vi "Periodic Tasks.vi"(8 "error constant":errorcluster) -> ()   [LabVIEW 2014]
doc: "This VI runs in parallel to other tasks. It can contain as many user-defined periodic loops as you need. These can carry out PID or other sorts of timed response."
uses:
  <vilib>/Rock Robotics/WPI/Relay/WPI_RelayValue.ctl
  <vilib>/Rock Robotics/WPI/Solenoid/WPI_SolenoidValue.ctl
  <vilib>/Rock Robotics/WPI/Compressor/WPI_CompressorGetSetRefNum.vi
  <vilib>/Rock Robotics/WPI/RobotDrive/WPI_RobotDriveGetSetRefNum.vi
  Robot Global Data.vi
  <vilib>/Rock Robotics/WPI/RobotDrive/WPI_RobotDriveMecanumDrive_Cartesian.vi
  <vilib>/addons/control/pid/pid.llb/PID (DBL).vi
  navX-MXP Library/navX-MXP IMU.lvlib
  <vilib>/addons/control/pid/NI_PID_pid.lvlib
panel:
  out "Voltage 2":dbl
  out "Level Pre Coerce":sgl
  out "String Potentiometer":dbl
  out "Setpoint from Teleop":dbl(slide) scale=3.7..4.5
  in  "SetPoint":dbl(slide) step=0.01 scale=3.7..4.5
  out "Brake":bool
  out "Doors Oper":bool
  out "Grabber":bool
  out "output":dbl format="%.2f"
  out "Voltage":dbl(slide) scale=0.0..5.0
  in  "proportional gain (Kc)":dbl=10.0 step=0.01
  in  "integral time (Ti, min)":dbl=0.001 step=0.01
  in  "derivative time (Td, min)":dbl=0.001 step=0.01
  in  "dt (s)":dbl=-1.0 format="%.3f"
  out "Lifter":bool
  out "Rotation":dbl
  out "Y":dbl
  out "X":dbl
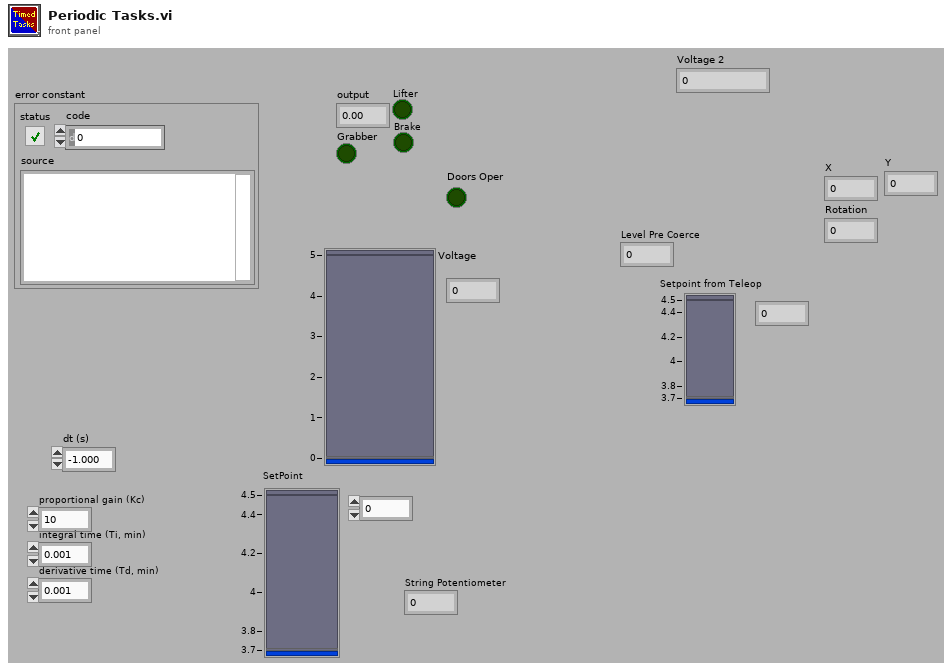
[diagram p1: front panel]
types:
  T1 = typedef "navX-MXP IMU.lvlib/navX SPI DevRef.ctl" = cluster{"SPIDevRef":T2, "Board Information":T5, "Status":T6, "Offsets":cluster{"Yaw":dbl, "Quat W":dbl, "Quat X":dbl, "Quat Y":dbl, "Quat Z":dbl}, "Update Rate (4Hz-60Hz)":u8, "refnum name":string, "error":errorcluster}
  T2 = typedef "WPI_SPIDevRef.ctl" = cluster{"DevStatus":errorcluster, "Handle":i32, "Controller":T3, "SPI Bus":T4}
  T3 = typedef "FPGA_TypedefDigitalModule.ctl" = enum16{"Controller 1"}
  T4 = typedef "spi_bus.ctl" = enum16{"SPI On-Board, CS0", "SPI On-Board, CS1", "SPI On-Board, CS2", "SPI On-Board, CS3", "SPI MXP", "Invalid"}
  T5 = typedef "navX-MXP IMU.lvlib/navX Board Information.ctl" = cluster{"WhoAmI (50 | 0x32)":u8, "Board Revision":u8, "Firmware Major Version":u8, "Firmware Minor Version":u8}
  T6 = typedef "navX-MXP IMU.lvlib/navX Status Data.ctl" = cluster{"Update Rate Hz":u8, "Accelerometer Full-Scale Range":u8, "Gyro Full-Scale Range":u16, "NAVX_OP_STATUS":T7, "NAVX_CAL_STATUS":T8, "NAVX_SELFTEST_STATUS":u8, "NAVX_SENSOR_STATUS":T9}
  T7 = typedef "navX-MXP IMU.lvlib/navX NAVX_OP_STATUS.ctl" = u8
  T8 = typedef "navX-MXP IMU.lvlib/navX NAVX_CAL_STATUS.ctl" = u8
  T9 = typedef "navX-MXP IMU.lvlib/navX NAVX_SENSOR_STATUS.ctl" = cluster{"MOVING":bool, "YAW_STABLE":bool, "MAG_DISTURBANCE":bool, "ALTITUDE_VALID":bool, "SEALEVEL_PRESS_SET":bool, "FUSED_HEADING_VALID":bool}
  T10 = typedef "navX-MXP IMU.lvlib/navX YPRH Data.ctl" = cluster{"Yaw":dbl, "Pitch":dbl, "Roll":dbl, "Heading":dbl}
  T11 = typedef "WPI_SolenoidValue.ctl" = enum16{"Off", "On", "Forward", "Reverse"}
  T12 = cluster{"proportional gain (Kc)":dbl, "integral time (Ti, min)":dbl, "derivative time (Td, min)":dbl}
  T13 = typedef "WPI_MotorControlDeviceRef.ctl" = cluster{"DeviceStatus":errorcluster, "Type":T14, "PWM":cluster{"Controller":T3, "PWM Channel":T15, "DeadBand":T16}, "CAN":cluster{"Device Number":u8, "Control Mode":T17, "Semaphore":T18, "Max Vout":dbl, "TalonSRX Control Mode":T19}, "Invert":bool, "TransformRef":T20, "InvTransformRef":T20}
  T14 = typedef "WPI_MotorControlType.ctl" = enum16{"PWM", "CAN", "CANTalonSRX"}
  T15 = typedef "FPGA_DIOPWMChannel.ctl" = enum8{"PWM 0", "PWM 1", "PWM 2", "PWM 3", "PWM 4", "PWM 5", "PWM 6", "PWM 7", "PWM 8", "PWM 9", "PWM MXP 0", "PWM MXP 1", "PWM MXP 2", "PWM MXP 3", "PWM MXP 4", "PWM MXP 5", "PWM MXP 6", "PWM MXP 7", "PWM MXP 8", "PWM MXP 9", "Invalid"}
  T16 = typedef "WPI_PWMDeadband.ctl" = cluster{"Name":string, "maxPositivePwm":i32, "minPositivePwm":i32, "centerPwm":i32, "maxNegativePwm":i32, "minNegativePwm":i32, "angularRange":u16}
  T17 = typedef "WPI_CANJaguar_ControlMode.ctl" = enum8{"Percent VBus", "Current", "Speed", "Position", "Voltage"}
  T18 = typedef "Semaphore RefNum" = refnum<k1>
  T19 = typedef "WPI_CANTalonSRX_APIControlMode.ctl" = enum8{"Percent VBus", "Speed", "Position", "Slave", "Unchanged / Invalid"}
  T20 = typedef "WPI_PWMTransform_ConPane.ctl" = refnum<vi>
  T21 = typedef "WPI_SolenoidDevRef.ctl" = cluster{"DevStatus":errorcluster, "Pneumatics Control Module":u8, "Forward Solenoid Channel":T22, "Reverse Solenoid Channel":T22}
  T22 = typedef "WPI_SolenoidChannel.ctl" = enum8{"Solenoid 0", "Solenoid 1", "Solenoid 2", "Solenoid 3", "Solenoid 4", "Solenoid 5", "Solenoid 6", "Solenoid 7", "Invalid"}
  T23 = typedef "WPI_AnalogChannelDevRef.ctl" = cluster{"DevStatus":errorcluster, "Controller":T24, "Analog Channel":T25}
  T24 = typedef "FPGA_TypedefAnalogModule.ctl" = enum16{"Controller 1"}
  T25 = typedef "FPGA_AIChannel.ctl" = enum8{"AI 0", "AI 1", "AI 2", "AI 3", "AI MXP 0", "AI MXP 1", "AI MXP 2", "AI MXP 3", "Invalid"}
  T26 = cluster{"Motor Speed":dbl, "Grabber":bool, "Go Up a Level":bool, "Go Down a Level":bool}
  T27 = cluster{"String Potentiometer":dbl, "Setpoint":dbl, "Level":sgl}
  T28 = typedef "WPI_RobotDriveDevRef.ctl" = cluster{"DevStatus":errorcluster, "Motors[]":T13[], "Square Inputs":bool, "Max Output":dbl}
  T29 = typedef "WPI_CompressorDevRef.ctl" = cluster{"DevStatus":errorcluster, "Pneumatics Control Module":u8}
  T30 = typedef "WPI_RelayDevRef.ctl" = cluster{"DevStatus":errorcluster, "Relay Channel":T31, "Controller":T3, "Relay Direction":T32}
  T31 = typedef "FPGA_DIORelayChannel.ctl" = enum8{"Relay 0", "Relay 1", "Relay 2", "Relay 3", "Invalid"}
  T32 = typedef "WPI_RelayDirection.ctl" = enum16{"Both directions", "Forward only", "Reverse only"}
  T33 = typedef "WPI_DigitalInputDevRef.ctl" = cluster{"DevStatus":errorcluster, "DIO Channel":T34, "Controller":T3}
  T34 = typedef "FPGA_DIOChannel.ctl" = enum8{"DIO 0", "DIO 1", "DIO 2", "DIO 3", "DIO 4", "DIO 5", "DIO 6", "DIO 7", "DIO 8", "DIO 9", "DIO MXP 0", "DIO MXP 1", "DIO MXP 2", "DIO MXP 3", "DIO MXP 4", "DIO MXP 5", "DIO MXP 6", "DIO MXP 7", "DIO MXP 8", "DIO MXP 9", "DIO MXP 10", "DIO MXP 11", "DIO MXP 12", "DIO MXP 13", "DIO MXP 14", "DIO MXP 15", "Invalid"}
  T35 = typedef "WPI_RelayValue.ctl" = enum16{"Off", "On", "Forward", "Reverse"}
  T36 = cluster{"Lifter Down":bool, "Right Infeed":enum16{"Off", "Forward", "Reverse"}, "Left Infeed":enum16{"Off", "Forward", "Reverse"}}
  T37 = cluster{"Front Right Motor":dbl, "Front Left Motor":dbl, "Rear Right Motor":dbl, "Rear Left Motor":dbl, "Current Heading":dbl, "Tote lift Up":bool, "Feeders Running":bool, "Pressure In Tank":dbl, "Image Data":string}
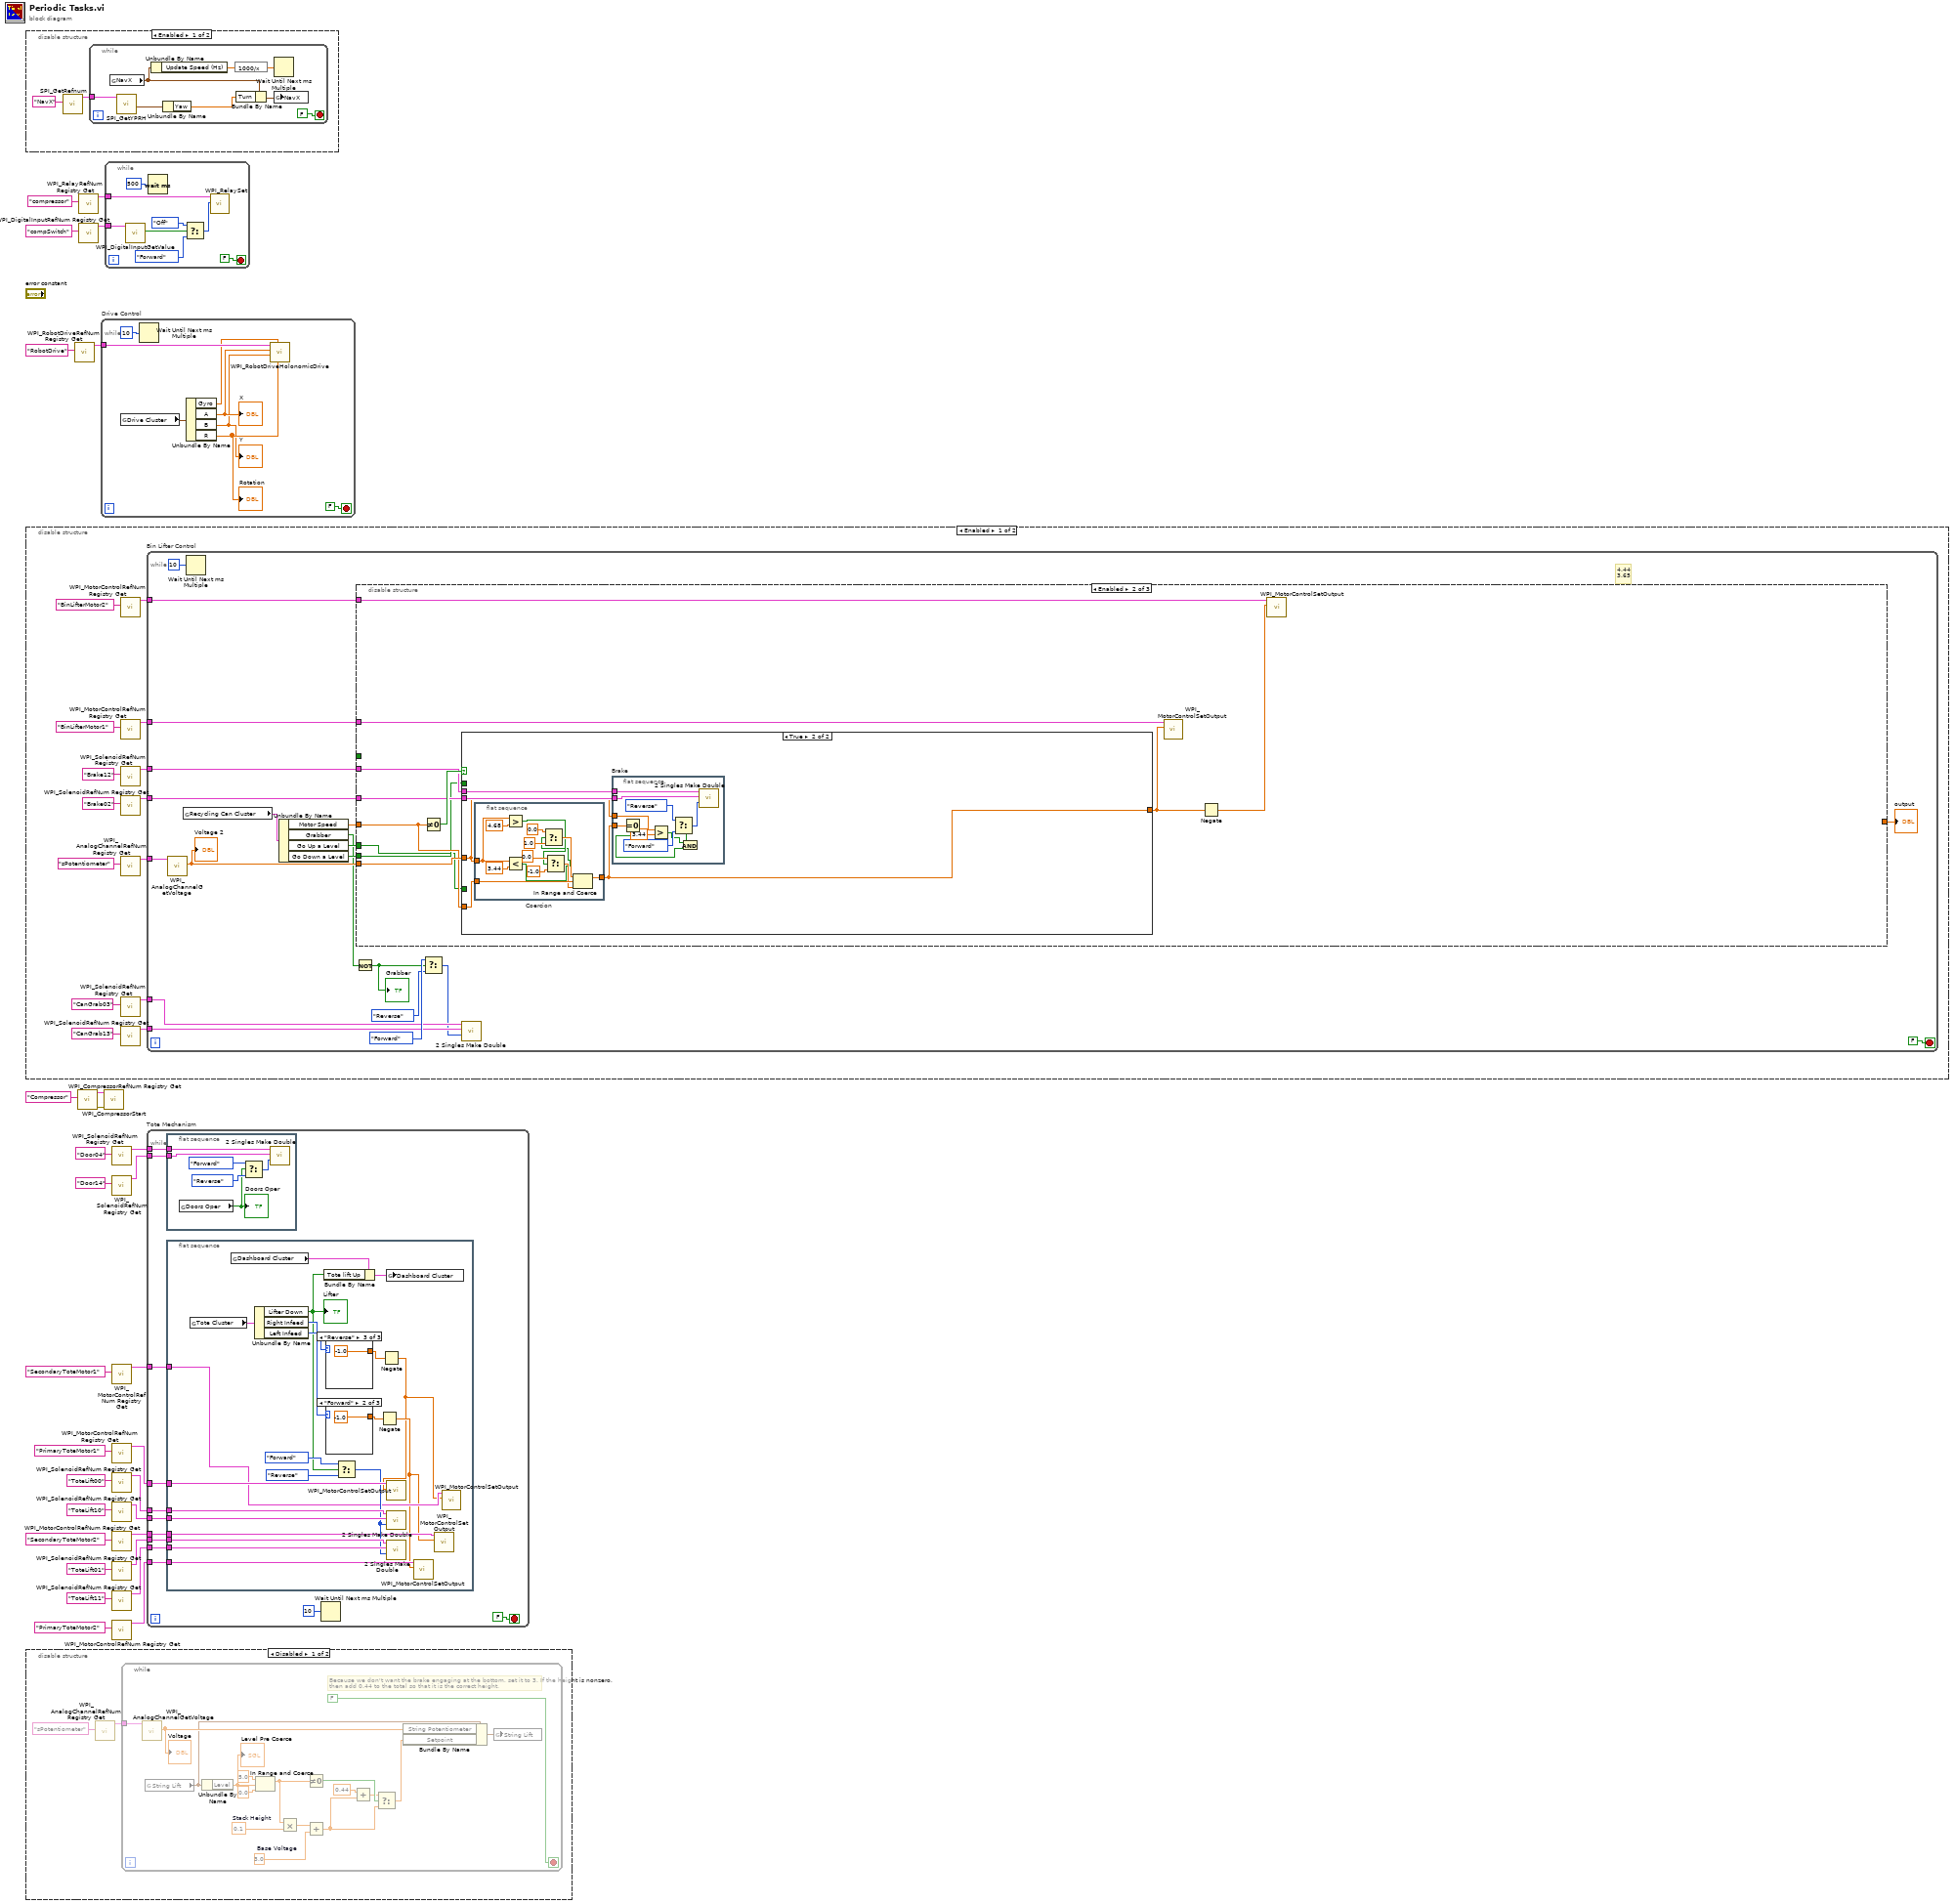
[diagram p0: block diagram]
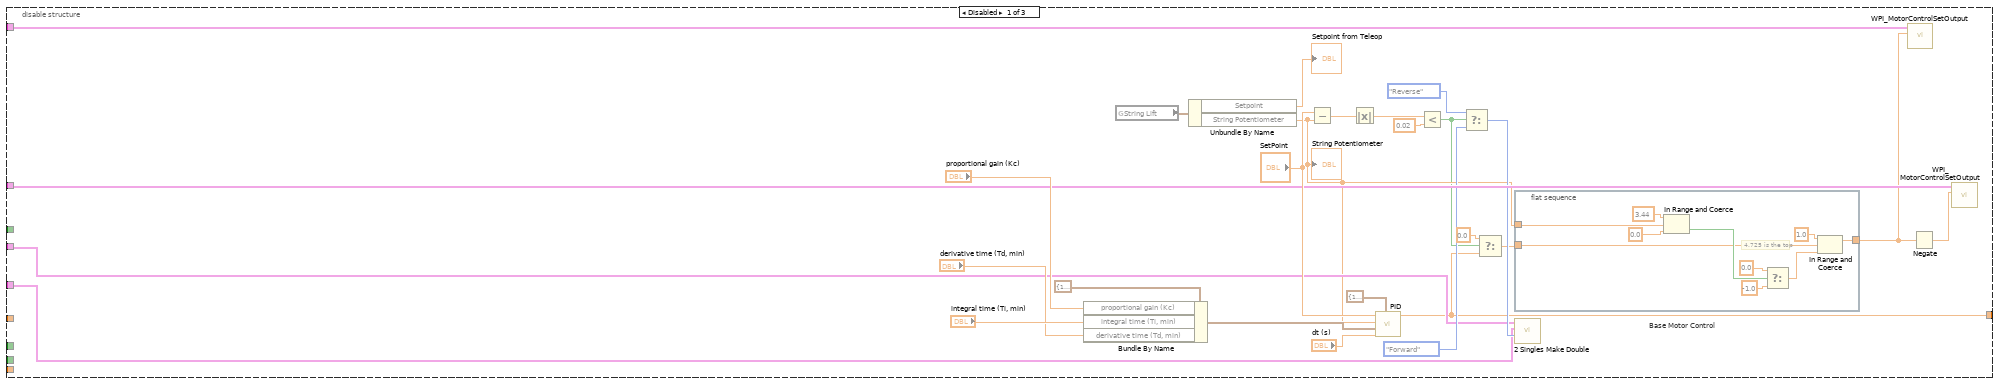
[diagram p2: hidden frame]
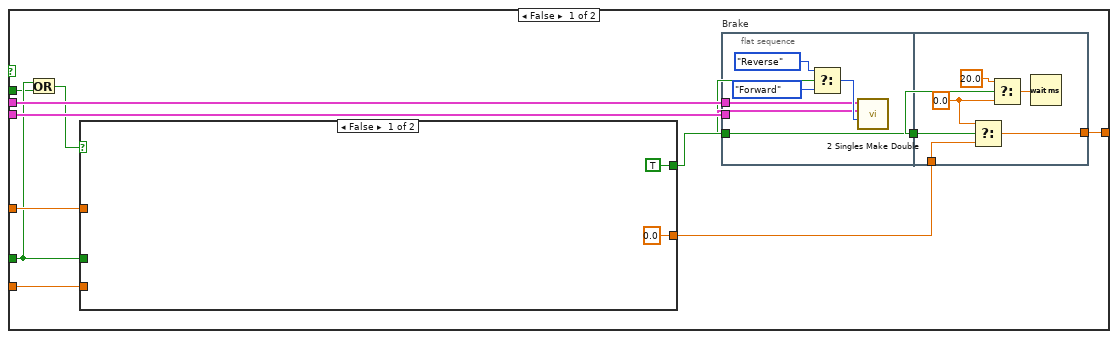
[diagram p3: hidden frame]
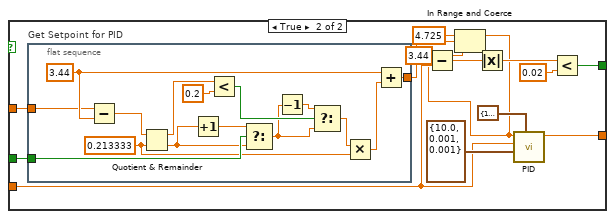
[diagram p4: hidden frame]
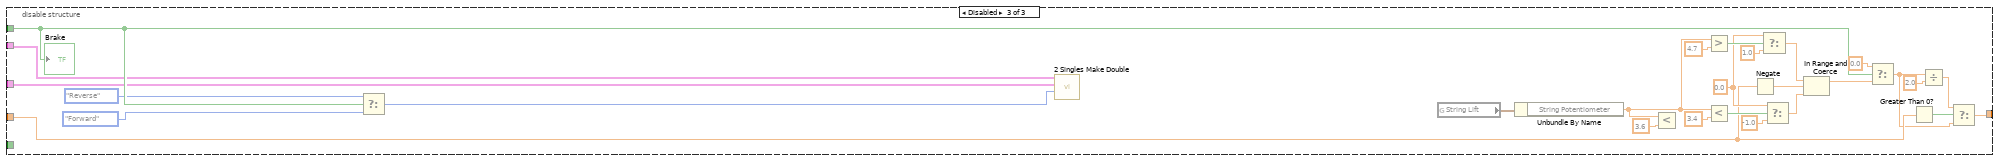
[diagram p5: hidden frame]
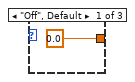
[diagram p9: hidden frame]
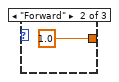
[diagram p10: hidden frame]
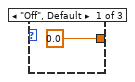
[diagram p11: hidden frame]
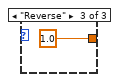
[diagram p12: hidden frame]
diagram:
  n1 = disable-structure shown="Enabled" {
    frame Enabled {
      n2 = call "SPI_GetRefnum.vi"("refnum name"="NavX") -> ("navX DevRef"=w30:T1)  [unwired: 9 in, 1 out]
      n3 = while {
        tunnel: w30 -> [w38]
        stop <- FALSE stop-if-true
        n4 = global read "Robot Global Data.vi" "NavX"() -> (w36:cluster{"Update Speed (Hz)":dbl, "Turn":dbl})
        n5 = call "SPI_GetYPRH.vi"("navX DevRef"=w38) -> ("YPRH"=w33:T10)  [unwired: 8 in, 2 out]
        n6 = Unbundle By Name(w36) -> ("Update Speed (Hz)"=w35:dbl)
        n7 = Unbundle By Name(w33) -> ("Yaw"=w32:dbl)
        n8 = expression code="1000/x"(w35) -> (w34:dbl)
        n9 = Bundle By Name(cluster=w36, "Turn"=w32) -> (w37:cluster{"Update Speed (Hz)":dbl, "Turn":dbl})
        n10 = Wait Until Next ms Multiple(millisecond multiple=w34) -> ()  [unwired: 1 out]
        n11 = global write "Robot Global Data.vi" "NavX"(w37) -> ()
      }
    }
    frame Disabled {
    }
  }
  n12 = disable-structure shown="Enabled" {
    frame Enabled {
      n13 = call <vilib>:"WPI_MotorControlRefNum Registry Get.vi"("refnum name"="BinLifterMotor2") -> ("MotorControlDevRef"=w52:T13)  [unwired: 9 in, 1 out]
      n14 = call <vilib>:"WPI_MotorControlRefNum Registry Get.vi"("refnum name"="BinLifterMotor1") -> ("MotorControlDevRef"=w50:T13)  [unwired: 9 in, 1 out]
      n15 = call <vilib>:"WPI_SolenoidRefNum Registry Get.vi"("refnum name"="Brake12") -> ("SolenoidDevRef"=w42:T21)  [unwired: 9 in, 1 out]
      n16 = call <vilib>:"WPI_SolenoidRefNum Registry Get.vi"("refnum name"="Brake02") -> ("SolenoidDevRef"=w44:T21)  [unwired: 9 in, 1 out]
      n17 = call <vilib>:"WPI_AnalogChannelRefNum Registry Get.vi"("refnum name"="sPotentiometer") -> ("AIDeviceRef"=w40:T23)  [unwired: 9 in, 1 out]
      n18 = call <vilib>:"WPI_SolenoidRefNum Registry Get.vi"("refnum name"="CanGrab03") -> ("SolenoidDevRef"=w46:T21)  [unwired: 9 in, 1 out]
      n19 = call <vilib>:"WPI_SolenoidRefNum Registry Get.vi"("refnum name"="CanGrab13") -> ("SolenoidDevRef"=w48:T21)  [unwired: 9 in, 1 out]
      n20 = while "Bin Lifter Control" {
        tunnel: w52 -> [w60]
        tunnel: w50 -> [w61]
        tunnel: w48 -> [w67]
        tunnel: w46 -> [w68]
        tunnel: w44 -> [w64]
        tunnel: w42 -> [w62]
        tunnel: w40 -> [w59]
        stop <- FALSE stop-if-true
        # "4.44\n3.65"
        n21 = call <vilib>:"WPI_AnalogChannelGetVoltage.vi"("AIDeviceRef"=w59) -> ("Voltage"=w58:dbl)  [unwired: 8 in, 2 out]
        "Voltage 2" <- w58
        n22 = global read "Robot Global Data.vi" "Recycling Can Cluster"() -> (w72:T26)
        n23 = Wait Until Next ms Multiple(millisecond multiple=u32 10) -> ()  [unwired: 1 out]
        n24 = Unbundle By Name(w72) -> ("Motor Speed"=w65:dbl, "Grabber"=w55:bool, "Go Up a Level"=w56:bool, "Go Down a Level"=w57:bool)
        n25 = Not(x=w55) -> (.not. x?=w54:bool)
        "Grabber" <- w54
        n26 = disable-structure shown="Enabled" {
          disable-tunnel: [w79 _ w212] -> w63
          disable-tunnel: w65 -> [_ w119 w215]
          disable-tunnel: _ -> [_ _ w220]
          disable-tunnel: w64 -> [w81 w117 w211]
          disable-tunnel: w62 -> [w82 w118 w208]
          disable-tunnel: w61 -> [w87 w116 _]
          disable-tunnel: w60 -> [w86 w115 _]
          disable-tunnel: w58 -> [_ w121 _]
          disable-tunnel: w57 -> [_ w114 _]
          disable-tunnel: w56 -> [_ w113 _]
          frame Disabled {
            n27 = Bundle By Name(cluster=T12 {"proportional gain (Kc)"=1.0, "integral time (Ti, min)"=0.01, "derivative time (Td, min)"=0.0} ("PID gains"), "proportional gain (Kc)"="proportional gain (Kc)", "integral time (Ti, min)"="integral time (Ti, min)", "derivative time (Td, min)"="derivative time (Td, min)") -> (w99:T12)
            n28 = global read "Robot Global Data.vi" "String Lift"() -> (w93:T27)
            n29 = Unbundle By Name(w93) -> ("Setpoint"=→"Setpoint from Teleop":dbl, "String Potentiometer"=w80:dbl)
            "String Potentiometer" <- w80
            n30 = Subtract(x="SetPoint", y=w80) -> (x-y=w90:dbl)
            n31 = Absolute Value(x=w90) -> (abs(x)=w75:dbl)
            n32 = call-poly <vilib>:"PID.vi"("output range"=cluster{"output high":dbl, "output low":dbl} {"output high"=1.0, "output low"=-1.0}, "dt (s)"="dt (s)", "PID gains"=w99, "process variable"=w80, "setpoint"="SetPoint") -> ("output"=w79:dbl)  [unwired: 5 in, 1 out]
            n33 = Less?(x=w75, y=0.02) -> (x < y?=w74:bool)
            n34 = Select(t=WPI_SolenoidValue."Reverse" ("Value"), s=w74, f=WPI_SolenoidValue."Forward" ("Value")) -> (s? t:f=w85:T11)
            n35 = Select(t=0.0, s=w74, f=w79) -> (s? t:f=w78:dbl)
            n36 = flat-sequence "Base Motor Control" {
              tunnel: w80 -> [w108]
              tunnel: w78 -> [w102]
              tunnel: [w101] -> w77
              frame #0 {
                # "4.725 is the top"
                n37 = In Range and Coerce(upper limit=3.44, x=w108, lower limit=0.0) -> (In Range?=w106:bool)  [unwired: 1 out]
                n38 = Select(t=0.0, s=w106, f=-1.0) -> (s? t:f=w105:dbl)
                n39 = In Range and Coerce(upper limit=1.0, x=w102, lower limit=w105) -> (coerced(x)=w101:dbl)  [unwired: 1 out]
              }
            }
            n40 = call "2 Singles Make Double.vi"("Value"=w85, "Reverse In"=w81, "Forward In"=w82) -> ()  [unwired: 7 in, 2 out]
            n41 = call <vilib>:"WPI_MotorControlSetOutput.vi"("Output"=w77, "MotorControlDevRef"=w86) -> ()  [unwired: 7 in, 3 out]
            n42 = Negate(x=w77) -> (-x=w76:dbl)
            n43 = call <vilib>:"WPI_MotorControlSetOutput.vi"("Output"=w76, "MotorControlDevRef"=w87) -> ()  [unwired: 7 in, 3 out]
          }
          frame Enabled {
            n44 = Not Equal To 0?(x=w119) -> (x != 0?=w120:bool)
            n45 = case shown="True" w120 {
              tunnel: w121 -> [w132 w176]
              tunnel: w119 -> [w131 w180]
              tunnel: w118 -> [w129 w179]
              tunnel: w117 -> [w128 w178]
              tunnel: [w125 w177] -> w111
              tunnel: w114 -> [w123 _]
              tunnel: w113 -> [w124 _]
              frame False {
                n46 = Or(x=w124, y=w123) -> (x .or. y?=w122:bool)
                n47 = case shown="False" w122 {
                  tunnel: w132 -> [_ w148]
                  tunnel: w124 -> [_ w147]
                  tunnel: w131 -> [_ w143]
                  tunnel: [TRUE w140] -> w130
                  tunnel: [0.0 ("output") w139] -> w126
                  frame False {
                  }
                  frame True {
                    n48 = flat-sequence "Get Setpoint for PID" {
                      tunnel: w148 -> [w158]
                      tunnel: w147 -> [w157]
                      tunnel: [w149] -> w138
                      frame #0 {
                        w151 = 0.213333 ("y")
                        w163 = 3.44 ("y")
                        n49 = Subtract(x=w158, y=w163) -> (x-y=w161:dbl)
                        n50 = Quotient & Remainder(x=w161, y=w151) -> (x-y*floor(x/y)=w160:dbl, floor(x/y)=w152:dbl)
                        n51 = Increment(x=w152) -> (x+1=w156:dbl)
                        n52 = Less?(x=w160, y=0.2) -> (x < y?=w155:bool)
                        n53 = Select(t=w156, s=w157, f=w152) -> (s? t:f=w153:dbl)
                        n54 = Decrement(x=w153) -> (x-1=w154:dbl)
                        n55 = Select(t=w154, s=w155, f=w153) -> (s? t:f=w150:dbl)
                        n56 = Multiply(x=w150, y=w151) -> (x*y=w162:dbl)
                        n57 = Add(x=w163, y=w162) -> (x+y=w149:dbl)
                      }
                    }
                    n58 = In Range and Coerce(upper limit=4.725, x=w138, lower limit=3.44) -> (coerced(x)=w135:dbl)  [unwired: 1 out]
                    n59 = Subtract(x=w135, y=w143) -> (x-y=w144:dbl)
                    n60 = Absolute Value(x=w144) -> (abs(x)=w142:dbl)
                    n61 = call-poly <vilib>:"PID.vi"("output range"=cluster{"output high":dbl, "output low":dbl} {"output high"=1.0, "output low"=-1.0}, "PID gains"=T12 {"proportional gain (Kc)"=10.0, "integral time (Ti, min)"=0.001, "derivative time (Td, min)"=0.001}, "process variable"=w143, "setpoint"=w135) -> ("output"=w139:dbl)  [unwired: 6 in, 1 out]
                    n62 = Less?(x=w142, y=0.02) -> (x < y?=w140:bool)
                  }
                }
                n63 = flat-sequence "Brake" {
                  tunnel: w129 -> [w166]
                  tunnel: w128 -> [w165]
                  tunnel: w130 -> [w164]
                  tunnel: [w164] -> w127
                  tunnel: w127 -> [w173]
                  tunnel: w126 -> [w175]
                  tunnel: [w174] -> w125
                  frame #0 {
                    n64 = Select(t=WPI_SolenoidValue."Reverse" ("Value"), s=w164, f=WPI_SolenoidValue."Forward" ("Value")) -> (s? t:f=w169:T11)
                    n65 = call "2 Singles Make Double.vi"("Value"=w169, "Reverse In"=w165, "Forward In"=w166) -> ()  [unwired: 7 in, 2 out]
                  }
                  frame #1 {
                    w172 = 0.0 ("t")
                    n66 = Select(t=w172, s=w173, f=w175) -> (s? t:f=w174:dbl)
                    n67 = Select(t=20.0, s=w173, f=w172) -> (s? t:f=w170:dbl)
                    n68 = Wait (ms)(milliseconds to wait=w170) -> ()  [unwired: 1 out]
                  }
                }
              }
              frame True {
                n69 = flat-sequence "Coercion" {
                  tunnel: w176 -> [w203]
                  tunnel: w180 -> [w201]
                  tunnel: [w195] -> w177
                  frame #0 {
                    n70 = Greater?(x=w203, y=4.68) -> (0:w193:bool)
                    n71 = Less?(x=w203, y=3.44) -> (x < y?=w192:bool)
                    n72 = Select(t=0.0, s=w192, f=1.0) -> (s? t:f=w200:dbl)
                    n73 = Select(t=0.0, s=w193, f=-1.0) -> (s? t:f=w199:dbl)
                    n74 = In Range and Coerce(upper limit=w200, x=w201, lower limit=w199) -> (coerced(x)=w195:dbl)  [unwired: 1 out]
                  }
                }
                n75 = flat-sequence "Brake" {
                  tunnel: w179 -> [w188]
                  tunnel: w178 -> [w187]
                  tunnel: w177 -> [w186]
                  tunnel: w176 -> [w185]
                  frame #0 {
                    n76 = Equal To 0?(x=w186) -> (x = 0?=w182:bool)
                    n77 = Greater?(x=w185, y=3.44) -> (0:w183:bool)
                    n78 = And(x=w183, y=w182) -> (x .and. y?=w181:bool)
                    n79 = Select(t=WPI_SolenoidValue."Reverse" ("Value"), s=w181, f=WPI_SolenoidValue."Forward" ("Value")) -> (s? t:f=w191:T11)
                    n80 = call "2 Singles Make Double.vi"("Value"=w191, "Reverse In"=w187, "Forward In"=w188) -> ()  [unwired: 7 in, 2 out]
                  }
                }
              }
            }
            n81 = call <vilib>:"WPI_MotorControlSetOutput.vi"("Output"=w111, "MotorControlDevRef"=w116) -> ()  [unwired: 7 in, 3 out]
            n82 = Negate(x=w111) -> (-x=w112:dbl)
            n83 = call <vilib>:"WPI_MotorControlSetOutput.vi"("Output"=w112, "MotorControlDevRef"=w115) -> ()  [unwired: 7 in, 3 out]
          }
          frame Disabled {
            w223 = 0.0 ("t")
            n84 = Select(t=WPI_SolenoidValue."Reverse" ("Value"), s=w220, f=WPI_SolenoidValue."Forward" ("Value")) -> (s? t:f=w205:T11)
            n85 = call "2 Singles Make Double.vi"("Value"=w205, "Reverse In"=w211, "Forward In"=w208) -> ()  [unwired: 7 in, 2 out]
            n86 = global read "Robot Global Data.vi" "String Lift"() -> (w231:T27)
            n87 = Unbundle By Name(w231) -> ("String Potentiometer"=w218:dbl)
            n88 = Less?(x=w218, y=3.6) -> ()  [unwired: 1 out]
            n89 = Greater?(x=w218, y=4.7) -> (0:w228:bool)
            n90 = Less?(x=w218, y=3.4) -> (x < y?=w225:bool)
            n91 = Negate(x=w215) -> (-x=w221:dbl)
            n92 = Select(t=w223, s=w228, f=1.0) -> (s? t:f=w227:dbl)
            n93 = Select(t=w223, s=w225, f=-1.0) -> (s? t:f=w226:dbl)
            n94 = In Range and Coerce(upper limit=w227, x=w221, lower limit=w226) -> (coerced(x)=w210:dbl)  [unwired: 1 out]
            n95 = Select(t=0.0, s=w220, f=w210) -> (s? t:f=w214:dbl)
            n96 = Greater Than 0?(x=w215) -> (x > 0?=w217:bool)
            n97 = Divide(x=w214, y=2.0) -> (x/y=w216:dbl)
            n98 = Select(t=w216, s=w217, f=w214) -> (s? t:f=w212:dbl)
            "Brake" <- w220
          }
        }
        "output" <- w63
        n99 = Select(t=WPI_SolenoidValue."Forward" ("Value"), s=w54, f=WPI_SolenoidValue."Reverse" ("Value")) -> (s? t:f=w66:T11)
        n100 = call "2 Singles Make Double.vi"("Value"=w66, "Reverse In"=w67, "Forward In"=w68) -> ()  [unwired: 7 in, 2 out]
      }
    }
    frame Disabled {
    }
  }
  n101 = disable-structure shown="Disabled" {
    frame Disabled {
      n102 = call <vilib>:"WPI_AnalogChannelRefNum Registry Get.vi"("refnum name"="sPotentiometer") -> ("AIDeviceRef"=w233:T23)  [unwired: 9 in, 1 out]
      n103 = while {
        tunnel: w233 -> [w249]
        stop <- FALSE stop-if-true
        w244 = 3.0  # Base Voltage
        w243 = 0.1  # Stack Height
        # "Because we don't want the brake engaging at the bottom, set it to 3. If the height is nonzero,\nthen add 0.44 to the total so that it is the correct height."
        n104 = call <vilib>:"WPI_AnalogChannelGetVoltage.vi"("AIDeviceRef"=w249) -> ("Voltage"=w247:dbl)  [unwired: 8 in, 2 out]
        "Voltage" <- w247
        n105 = global read "Robot Global Data.vi" "String Lift"() -> (w246:T27)
        n106 = Unbundle By Name(w246) -> ("Level"=w242:sgl)
        "Level Pre Coerce" <- w242
        n107 = In Range and Coerce(upper limit=sgl 5.0, x=w242, lower limit=sgl 0.0) -> (coerced(x)=w239:sgl)  [unwired: 1 out]
        n108 = Multiply(x=w239, y=w243) -> (x*y=w245:dbl)
        n109 = Not Equal To 0?(x=w239) -> (x != 0?=w238:bool)
        n110 = Add(x=w245, y=w244) -> (x+y=w236:dbl)
        n111 = Add(x=0.44, y=w236) -> (x+y=w237:dbl)
        n112 = Select(t=w237, s=w238, f=w236) -> (s? t:f=w234:dbl)
        n113 = Bundle By Name(cluster=w246, "String Potentiometer"=w247, "Setpoint"=w234) -> (w248:T27)
        n114 = global write "Robot Global Data.vi" "String Lift"(w248) -> ()
      }
    }
    frame Enabled {
    }
  }
  n115 = call <vilib>:"WPI_RobotDriveRefNum Registry Get.vi"("refnum name"="RobotDrive") -> ("RobotDriveDevRef"=w10:T28)  [unwired: 9 in, 1 out]
  n116 = call <vilib>:"WPI_CompressorRefNum Registry Get.vi"("refnum name"="Compressor") -> ("error out"=w24:errorcluster, "CompressorDevRef"=w25:T29)  [unwired: 9 in]
  n117 = call <vilib>:"WPI_RelayRefNum Registry Get.vi"("refnum name"="compressor") -> ("RelayDevRef"=w1:T30)  [unwired: 9 in, 1 out]
  n118 = call <vilib>:"WPI_DigitalInputRefNum Registry Get.vi"("refnum name"="compSwitch") -> ("DigitalInputDevRef"=w3:T33)  [unwired: 9 in, 1 out]
  n119 = while "Drive Control" {
    tunnel: w10 -> [w257]
    stop <- FALSE stop-if-true
    n120 = global read "Robot Global Data.vi" "Drive Cluster"() -> (w253:cluster{"A":dbl, "B":dbl, "R":dbl, "Gyro":dbl})
    n121 = Wait Until Next ms Multiple(millisecond multiple=u32 10) -> ()  [unwired: 1 out]
    n122 = Unbundle By Name(w253) -> ("Gyro"=w256:dbl, "A"=w254:dbl, "B"=w251:dbl, "R"=w252:dbl)
    "X" <- w254
    "Y" <- w251
    "Rotation" <- w252
    n123 = call-poly <vilib>:"WPI_RobotDriveHolonomicDrive.vi"("Rotation"=w252, "Gyro Angle"=w256, "Y"=w251, "X"=w254, "RobotDriveDevRef"=w257) -> ()  [unwired: 4 in, 3 out]
  }
  n124 = call <vilib>:"WPI_CompressorStart.vi"("error in (no error)"=w24, "CompressorDevRef"=w25) -> ()  [unwired: 8 in, 2 out]
  n125 = while {
    tunnel: w3 -> [w265]
    tunnel: w1 -> [w263]
    stop <- FALSE stop-if-true
    n126 = call <vilib>:"WPI_DigitalInputGetValue.vi"("DigitalInputDevRef"=w265) -> ("Value"=w261:bool)  [unwired: 8 in, 2 out]
    n127 = Wait (ms)(milliseconds to wait=u32 500) -> ()  [unwired: 1 out]
    n128 = Select(t=WPI_RelayValue."Off" ("RelayValue"), s=w261, f=WPI_RelayValue."Forward" ("RelayValue")) -> (s? t:f=w259:T35)
    n129 = call <vilib>:"WPI_RelaySet.vi"("RelayValue"=w259, "RelayDevRef"=w263) -> ()  [unwired: 8 in, 2 out]
  }
  n130 = call <vilib>:"WPI_SolenoidRefNum Registry Get.vi"("refnum name"="Door04") -> ("SolenoidDevRef"=w12:T21)  [unwired: 9 in, 1 out]
  n131 = call <vilib>:"WPI_SolenoidRefNum Registry Get.vi"("refnum name"="Door14") -> ("SolenoidDevRef"=w13:T21)  [unwired: 9 in, 1 out]
  n132 = call <vilib>:"WPI_MotorControlRefNum Registry Get.vi"("refnum name"="SecondaryToteMotor1") -> ("MotorControlDevRef"=w9:T13)  [unwired: 9 in, 1 out]
  n133 = call <vilib>:"WPI_MotorControlRefNum Registry Get.vi"("refnum name"="PrimaryToteMotor1") -> ("MotorControlDevRef"=w27:T13)  [unwired: 9 in, 1 out]
  n134 = call <vilib>:"WPI_SolenoidRefNum Registry Get.vi"("refnum name"="ToteLift00") -> ("SolenoidDevRef"=w22:T21)  [unwired: 9 in, 1 out]
  n135 = call <vilib>:"WPI_SolenoidRefNum Registry Get.vi"("refnum name"="ToteLift10") -> ("SolenoidDevRef"=w20:T21)  [unwired: 9 in, 1 out]
  n136 = call <vilib>:"WPI_MotorControlRefNum Registry Get.vi"("refnum name"="SecondaryToteMotor2") -> ("MotorControlDevRef"=w8:T13)  [unwired: 9 in, 1 out]
  n137 = call <vilib>:"WPI_SolenoidRefNum Registry Get.vi"("refnum name"="ToteLift01") -> ("SolenoidDevRef"=w17:T21)  [unwired: 9 in, 1 out]
  n138 = call <vilib>:"WPI_SolenoidRefNum Registry Get.vi"("refnum name"="ToteLift11") -> ("SolenoidDevRef"=w16:T21)  [unwired: 9 in, 1 out]
  n139 = call <vilib>:"WPI_MotorControlRefNum Registry Get.vi"("refnum name"="PrimaryToteMotor2") -> ("MotorControlDevRef"=w5:T13)  [unwired: 9 in, 1 out]
  n140 = while "Tote Mechanism" {
    tunnel: w22 -> [w272]
    tunnel: w5 -> [w277]
    tunnel: w27 -> [w276]
    tunnel: w20 -> [w271]
    tunnel: w17 -> [w270]
    tunnel: w16 -> [w269]
    tunnel: w13 -> [w273]
    tunnel: w12 -> [w274]
    tunnel: w9 -> [w268]
    tunnel: w8 -> [w267]
    stop <- FALSE stop-if-true
    n141 = flat-sequence {
      tunnel: w274 -> [w284]
      tunnel: w273 -> [w283]
      frame #0 {
        n142 = global read "Robot Global Data.vi" "Doors Oper"() -> (w280:bool)
        "Doors Oper" <- w280
        n143 = Select(t=WPI_SolenoidValue."Forward" ("Value"), s=w280, f=WPI_SolenoidValue."Reverse" ("Value")) -> (s? t:f=w279:T11)
        n144 = call "2 Singles Make Double.vi"("Value"=w279, "Reverse In"=w283, "Forward In"=w284) -> ()  [unwired: 7 in, 2 out]
      }
    }
    n145 = flat-sequence {
      tunnel: w277 -> [w302]
      tunnel: w276 -> [w301]
      tunnel: w272 -> [w297]
      tunnel: w271 -> [w296]
      tunnel: w270 -> [w293]
      tunnel: w269 -> [w292]
      tunnel: w268 -> [w290]
      tunnel: w267 -> [w289]
      frame #0 {
        n146 = global read "Robot Global Data.vi" "Tote Cluster"() -> (w305:T36)
        n147 = global read "Robot Global Data.vi" "Dashboard Cluster"() -> (w303:T37)
        n148 = Unbundle By Name(w305) -> ("Lifter Down"=w294:bool, "Right Infeed"=w300:enum16{"Off", "Forward", "Reverse"}, "Left Infeed"=w299:enum16{"Off", "Forward", "Reverse"})
        "Lifter" <- w294
        n149 = Bundle By Name(cluster=w303, "Tote lift Up"=w294) -> (w304:T37)
        n150 = case shown="\"Reverse\"" w299 {
          tunnel: [0.0 ("f") 1.0 ("f") -1.0 ("f")] -> w286
          frame "Off", Default {
          }
          frame "Forward" {
          }
          frame "Reverse" {
          }
        }
        n151 = case shown="\"Forward\"" w300 {
          tunnel: [0.0 ("f") -1.0 ("f") 1.0 ("f")] -> w288
          frame "Off", Default {
          }
          frame "Forward" {
          }
          frame "Reverse" {
          }
        }
        n152 = Select(t=WPI_SolenoidValue."Forward" ("Value"), s=w294, f=WPI_SolenoidValue."Reverse" ("Value")) -> (s? t:f=w291:T11)
        n153 = Negate(x=w288) -> (-x=w287:dbl)
        n154 = Negate(x=w286) -> (-x=w285:dbl)
        n155 = global write "Robot Global Data.vi" "Dashboard Cluster"(w304) -> ()
        n156 = call <vilib>:"WPI_MotorControlSetOutput.vi"("Output"=w285, "MotorControlDevRef"=w301) -> ()  [unwired: 7 in, 3 out]
        n157 = call "2 Singles Make Double.vi"("Value"=w291, "Reverse In"=w296, "Forward In"=w297) -> ()  [unwired: 7 in, 2 out]
        n158 = call "2 Singles Make Double.vi"("Value"=w291, "Reverse In"=w292, "Forward In"=w293) -> ()  [unwired: 7 in, 2 out]
        n159 = call <vilib>:"WPI_MotorControlSetOutput.vi"("Output"=w287, "MotorControlDevRef"=w302) -> ()  [unwired: 7 in, 3 out]
        n160 = call <vilib>:"WPI_MotorControlSetOutput.vi"("Output"=w287, "MotorControlDevRef"=w289) -> ()  [unwired: 7 in, 3 out]
        n161 = call <vilib>:"WPI_MotorControlSetOutput.vi"("Output"=w285, "MotorControlDevRef"=w290) -> ()  [unwired: 7 in, 3 out]
      }
    }
    n162 = Wait Until Next ms Multiple(millisecond multiple=u32 10) -> ()  [unwired: 1 out]
  }
